vi "UDP Data Link - Configuration Utilities - Set Configuration File.vi"(8 "error in (no error)":errorcluster, 9 "Export to File on Save":refnum<vi>, 10 "Export Path":refnum<vi>, 11 "Item Ref in":T1 format="%.0x") -> (0 "error out":errorcluster, 3 "Item Ref out":T1 format="%.0x")   [LabVIEW 2016, in "UDP-Custom-Device System Explorer.lvlib"]
doc: "Sets the <b>Export to File Status</b> and <b>Export File</b> based on their associated page properties."
uses:
  UDP-Custom-Device System Explorer.lvlib
  <vilib>/NI Veristand/Custom Device API/Custom Device Item Ref.ctl
  Shared/Constants.vi
  <vilib>/NI Veristand/Custom Device API/Get Item Property (Boolean).vi
  <vilib>/NI Veristand/Custom Device API/Get Item Property (Path).vi
  <vilib>/NI VeriStand/Custom Device API/Custom Device API.lvlib
  Shared/UDP-Custom-Device Shared.lvlib
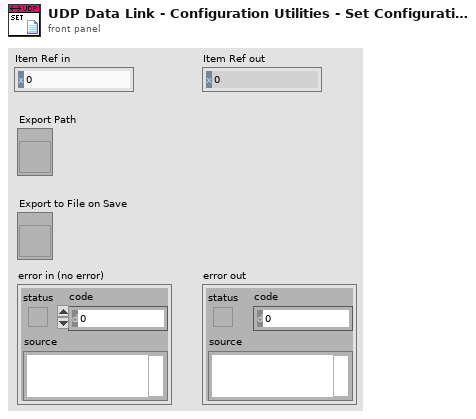
[diagram p1: front panel]
types:
  T1 = typedef "Custom Device API.lvlib/Custom Device Item Ref.ctl" = u64
  T2 = enum8{"Enabled", "Disabled", "Disabled and Grayed Out"}
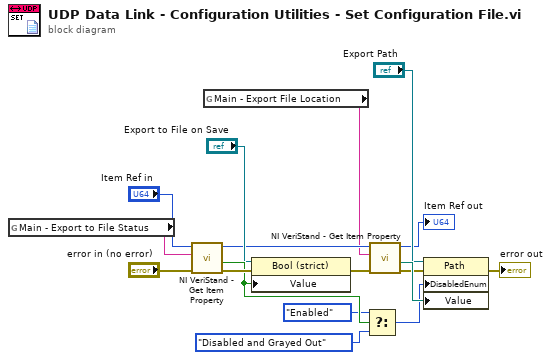
[diagram p0: block diagram]
diagram:
  n1 = global read "Constants.vi" "Main - Export to File Status"() -> (w2:string)
  n2 = call-poly <vilib>:"NI VeriStand - Get Item Property.vi"("error in (no error)"="error in (no error)", "Property Name"=w2, "Item Ref in"="Item Ref in") -> ("error out"=w16:errorcluster, "Value"=w11:bool, "Item Ref out"=w5:T1)  [unwired: 5 in, 1 out]
  n3 = global read "Constants.vi" "Main - Export File Location"() -> (w1:string)
  n4 = property class="Bool (strict)"(reference="Export to File on Save", error in=w16, "Value"=w11) -> (error out=w17:errorcluster)  [unwired: 1 out]
  n5 = Select(t=T2."Enabled" ("Disabled"), s=w11, f=T2."Disabled and Grayed Out" ("Disabled")) -> (s? t:f=w12:T2)
  n6 = call-poly <vilib>:"NI VeriStand - Get Item Property.vi"("error in (no error)"=w17, "Property Name"=w1, "Item Ref in"=w5) -> ("error out"=w13:errorcluster, "Value"=w15:path, "Item Ref out"=→"Item Ref out":T1)  [unwired: 5 in, 1 out]
  n7 = property class="Path"(reference="Export Path", error in=w13, "DisabledEnum"=w12, "Value"=w15) -> (error out=→"error out":errorcluster)  [unwired: 1 out]
